vi "LJStreamM stream data.vi"(0 "Data File Reference In":path, 1 "Handle In":i32, 2 "Channel Setup":T1={"Name"=["AIN0", "AIN1", "AIN2", "AIN3", "AIN4", "AIN5", "AIN6", "AIN7", "AIN8", "AIN9", "AIN10", "AIN11", "AIN12", "AIN13", "AIN14", "AIN15", "AIN16", "AIN17", "AIN18", "AIN19", "AIN20", "AIN21", "AIN22", "AIN23", "AIN24", "AIN25", "AIN26", "AIN27", "AIN28", "AIN29", "AIN30", "AIN31", "AIN32", "AIN33", "AIN34", "AIN35", "AIN36", "AIN37", "AIN38", "AIN39", "AIN40", "AIN41", "AIN42", "AIN43", "AIN44", "AIN45", "AIN46", "AIN47", "AIN48", "AIN49", "AIN50", "AIN51", "AIN52", "AIN53", "AIN54", "AIN55", "AIN56", "AIN57", "AIN58", "AIN59", "AIN60", "AIN61", "AIN62", "AIN63", "AIN64", "AIN65", "AIN66", "AIN67", "AIN68", "AIN69", "AIN70", "AIN71", "AIN72", "AIN73", "AIN74", "AIN75", "AIN76", "AIN77", "AIN78", "AIN79", "AIN80", "AIN81", "AIN82", "AIN83", "AIN84", "AIN85", "AIN86", "AIN87", "AIN88", "AIN89", "AIN90", "AIN91", "AIN92", "AIN93", "AIN94", "AIN95", "AIN96", "AIN97", "AIN98", "AIN99"], "", "Scaling Equation"=["y=a", "y=b", "y=c", "y=d", "y=e", "y=f", "y=g", "y=h", "y=i", "y=j", "y=k", "y=l", "y=m", "y=n", "y=o", "y=p", "y=q", "y=r", "y=s", "y=t", "y=u", "y=v", "y=w", "y=x", "y=y", "y=z", "y=a2", "y=b2", "y=c2", "y=d2", "y=e2", "y=f2", "y=g2", "y=h2", "y=i2", "y=j2", "y=k2", "y=l2", "y=m2", "y=n2", "y=o2", "y=p2", "y=q2", "y=r2", "y=s2", "y=t2", "y=u2", "y=v2", "y=w2", "y=x2", "y=y2", "y=z2", "y=a3", "y=b3", "y=c3", "y=d3", "y=e3", "y=f3", "y=g3", "y=h3", "y=i3", "y=j3", "y=k3", "y=l3", "y=m3", "y=n3", "y=o3", "y=p3", "y=q3", "y=r3", "y=s3", "y=t3", "y=u3", "y=v3", "y=w3", "y=x3", "y=y3", "y=z3", "y=a4", "y=b4", "y=c4", "y=d4", "y=e4", "y=f4", "y=g4", "y=h4", "y=i4", "y=j4", "y=k4", "y=l4", "y=m4", "y=n4", "y=o4", "y=p4", "y=q4", "y=r4", "y=s4", "y=t4", "y=u4", "y=v4"], "", "Graph?"=[TRUE, TRUE, TRUE, TRUE, FALSE, FALSE, FALSE, FALSE, FALSE, FALSE, FALSE, FALSE, FALSE, FALSE, FALSE, FALSE]}, 3 "# Channels":i32=1 min=1, 4 "Starting Scan Number":dbl, 5 "Scan Rate":dbl=100.0 format="%.3f", 7 "Error In":errorcluster, 8 "Data File Prefix":string="data", 9 "Disable Scaling*":bool=TRUE, 10 "Max File Size (Bytes)":i32=1048576 min=1 max=2000000000, 11 "Write To File":bool, 12 "Scans Per Read":i32, 14 "# Scans On Graph":i32=1000 min=0, 18 "Starting #":u32) -> (19 "Data File #":u32, 20 "Data File Reference Out":path=path "none", 21 "Handle Out":i32, 22 "Raw Value":dbl[](array[numeric]) format="%.6f", 23 "Scaled Value":dbl[](array[numeric]) format="%.6f", 24 "Waveform Graph":cluster{dbl, dbl, dbl[][]}(graph)={0.0, 0.0025, []}, 25 "LJMScanBacklog":dbl format="%.2f", 26 "DeviceScanBacklog":dbl format="%.2f", 27 "Error Out":errorcluster)   [LabVIEW 2026]
uses:
  Common Logger Controls/Channel Setup.ctl
  Common Logger VIs/LJM logger Globals.vi
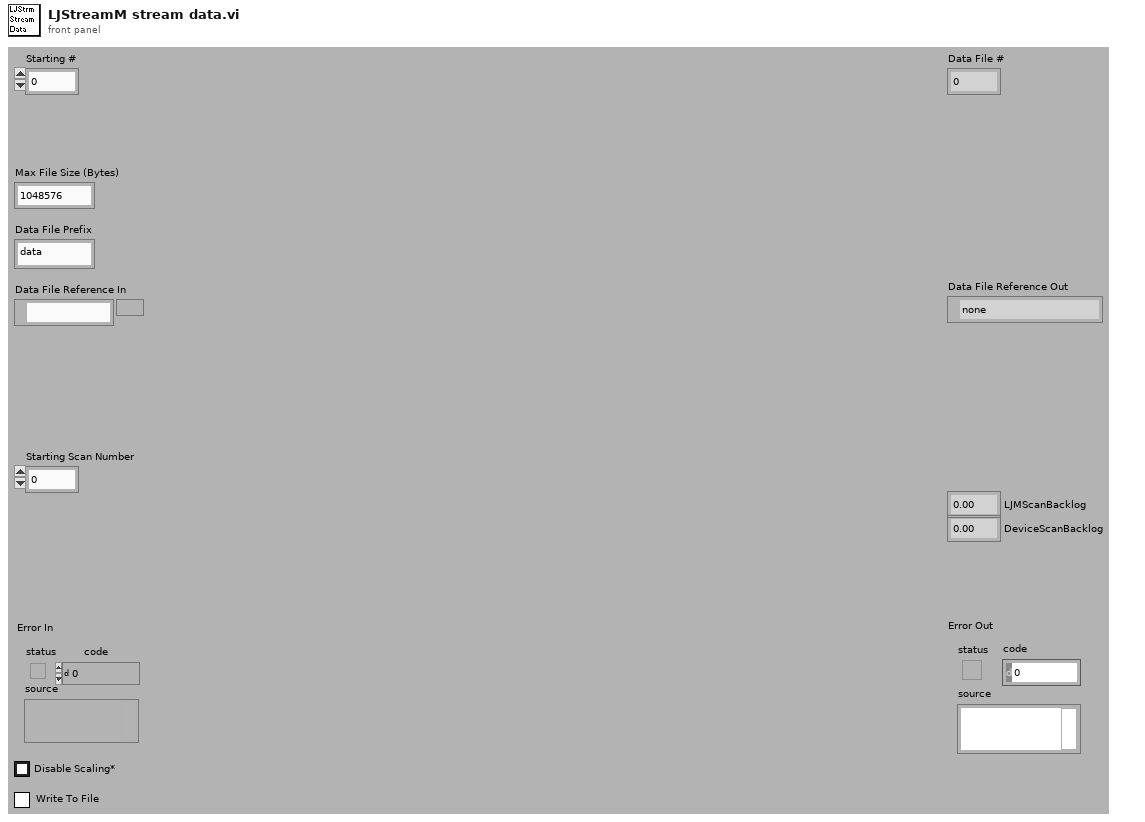
[diagram p1: front panel]
types:
  T1 = typedef "Channel Setup.ctl" = cluster{"Name":string[], string, "Scaling Equation":string[], string, "Graph?":bool[]}
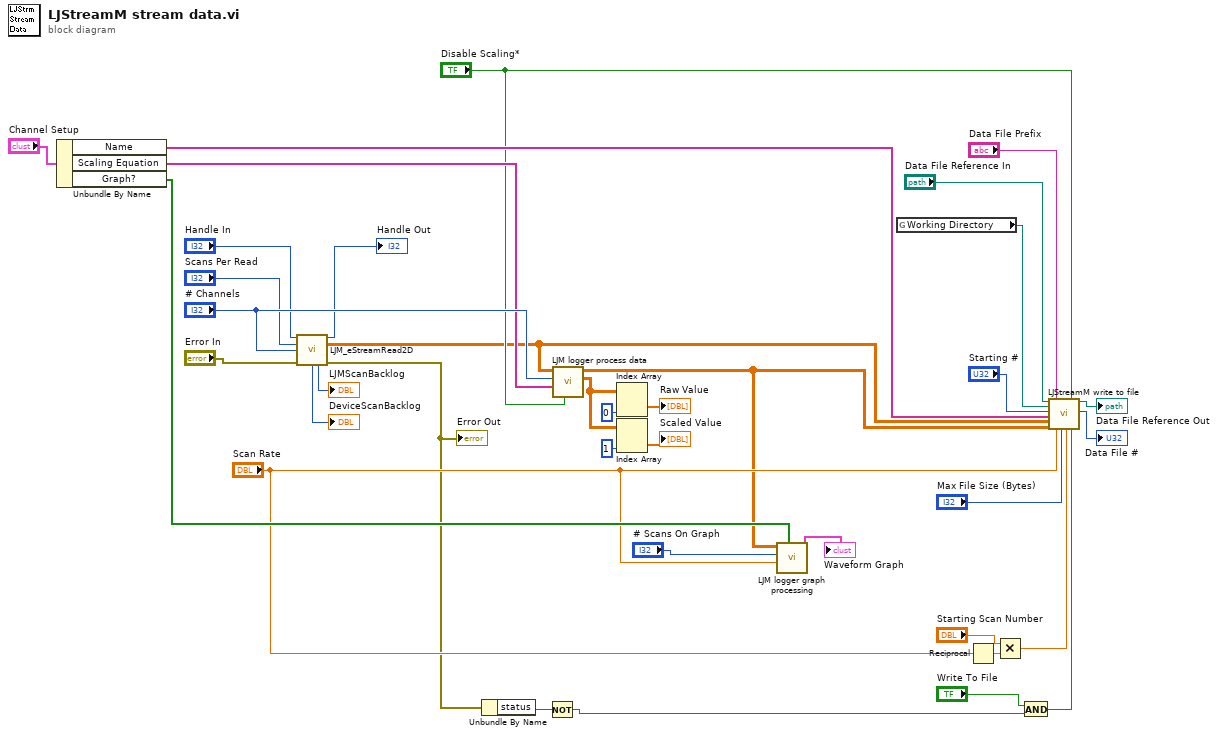
[diagram p0: block diagram]
diagram:
  n1 = Unbundle By Name("Channel Setup") -> ("Name"=w35:string[], "Scaling Equation"=w34:string[], "Graph?"=w33:bool[])
  n2 = call "LJM_eStreamRead2D.vi"("Handle In"="Handle In", "ScansPerRead"="Scans Per Read", "NumAddresses"="# Channels", "error in"="Error In") -> ("Handle Out"=→"Handle Out":i32, "aData Out"=w5:dbl[][], "DeviceScanBacklog"=→"DeviceScanBacklog":i32, "LJMScanBacklog"=→"LJMScanBacklog":i32, "error out"=w30:errorcluster)  [unwired: 7 in]
  "Error Out" <- w30
  n3 = Unbundle By Name(w30) -> ("status"=w3:bool)
  n4 = Not(x=w3) -> (.not. x?=w2:bool)
  n5 = call "LJM logger process data.vi"("Disable Scaling"="Disable Scaling*", "Scaling Equation"=w34, "# Channels"="# Channels", "Voltages"=w5) -> ("Volts,Scaled Averages"=w13:dbl[][], "Scaled Data"=w4:dbl[][])  [unwired: 5 in, 1 out]
  n6 = Index Array(array=w13, index (col)=0 ("Disabled Index (col)")) -> (element=→"Raw Value":dbl[])  [unwired: 1 in]
  n7 = Index Array(array=w13, index (col)=1 ("Disabled Index (col)")) -> (element=→"Scaled Value":dbl[])  [unwired: 1 in]
  n8 = call "LJM logger graph processing.vi"("Graph?"=w33, "Scan Rate"="Scan Rate", "Graph History (# scans)"="# Scans On Graph", "Scaled Data"=w4) -> ("Graph Data"=→"Waveform Graph":cluster{dbl, dbl, dbl[][]})  [unwired: 7 in]
  n9 = global read "LJM logger Globals.vi" "Working Directory"() -> (w11:path)
  n10 = Reciprocal(x="Scan Rate") -> (1/x=w17:dbl)
  n11 = Multiply(x="Starting Scan Number", y=w17) -> (x*y=w7:dbl)
  n12 = And(x="Write To File", y=w2) -> (x .and. y?=w8:bool)
  n13 = call "LJStreamM write to file.vi"("Data File Reference In"="Data File Reference In", "Working Directory"=w11, "Starting #"="Starting #", "Channel Names"=w35, "Raw Value"=w5, "Scaled Data"=w4, "Data File Prefix"="Data File Prefix", "Scan Rate"="Scan Rate", "Max File Size (Bytes)"="Max File Size (Bytes)", "Starting Scan Time"=w7, "Disable Scaling"="Disable Scaling*", "Write to file?"=w8) -> ("Data File Reference Out"=→"Data File Reference Out":path, "Data File #"=→"Data File #":u32)  [unwired: 5 in, 1 out]
